vi "N6701A_ReadCurrent.vi"(8 "error in (no error)":errorcluster, 10 "Channel Name (1)":string="2", 11 "VISA resource name":refnum<visa-resource-name>="PS2") -> (0 "error out":errorcluster, 2 "Measurement":dbl=-0.0009589195 format="%^.3e")   [LabVIEW 2015]
uses:
  <instrlib>/Agilent N6700 Series/Agilent N6700 Series.lvlib
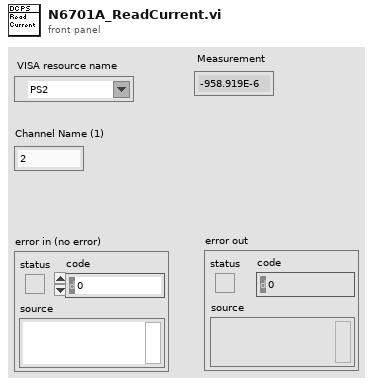
[diagram p1: front panel]
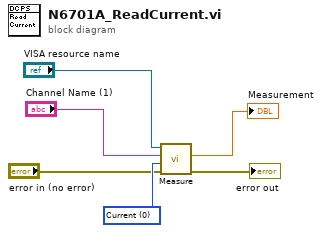
[diagram p0: block diagram]
diagram:
  w5 = 0 items=["Voltage"=1, "Current"=0] ("Measurement Type (1: Voltage)")
  n1 = call <instrlib>:"Measure.vi"("error in (no error)"="error in (no error)", "Measurement Type (1: Voltage)"=w5, "Channel Name (1)"="Channel Name (1)", "VISA resource name"="VISA resource name") -> ("error out"=→"error out":errorcluster, "Measurement"=→"Measurement":dbl)  [unwired: 5 in, 1 out]
